vi "test.vi"() -> ()   [LabVIEW 2013]
uses:
  InfoTable.lvclass
panel:
  out "数组":cluster{"ID":dbl, "食品名称":string, "价格":dbl}[](array[cluster])
  out "Exist?":bool
  out "食品信息 2":cluster{"ID":dbl, "食品名称":string, "价格":dbl}
  in  "食品信息":cluster{"ID":dbl, "食品名称":string, "价格":dbl}
  in  "枚举":enum16{"获取", "清空", "插入", "删除", "查询"}(ring)
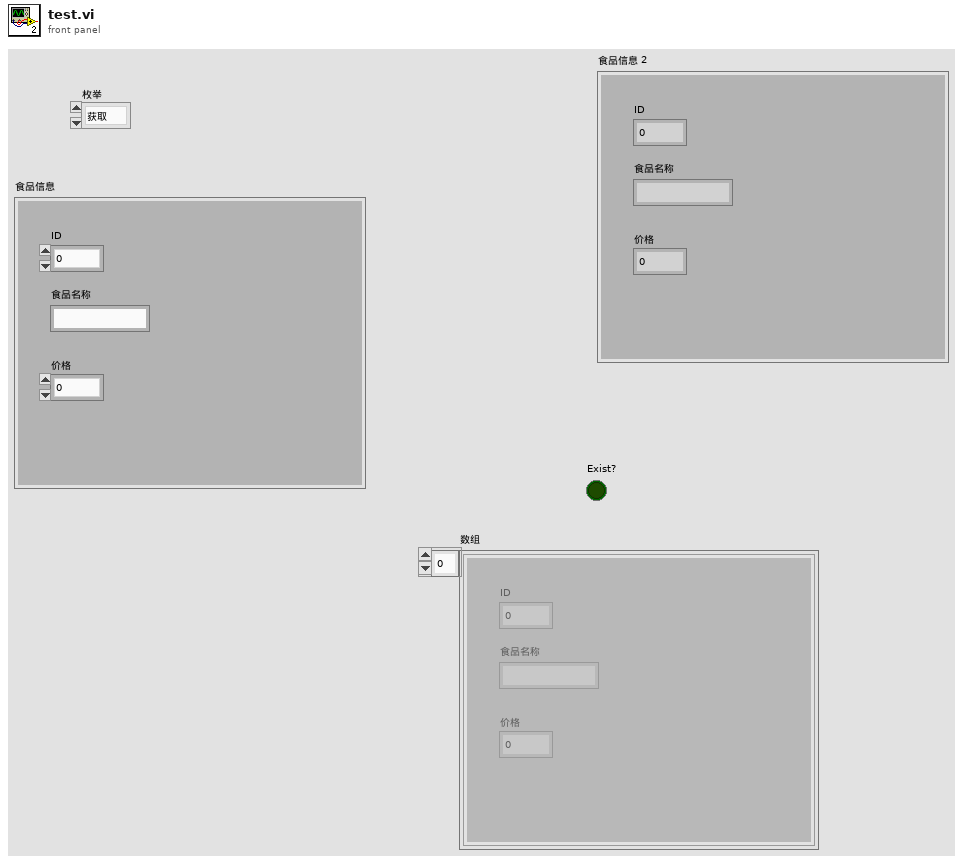
[diagram p1: front panel]
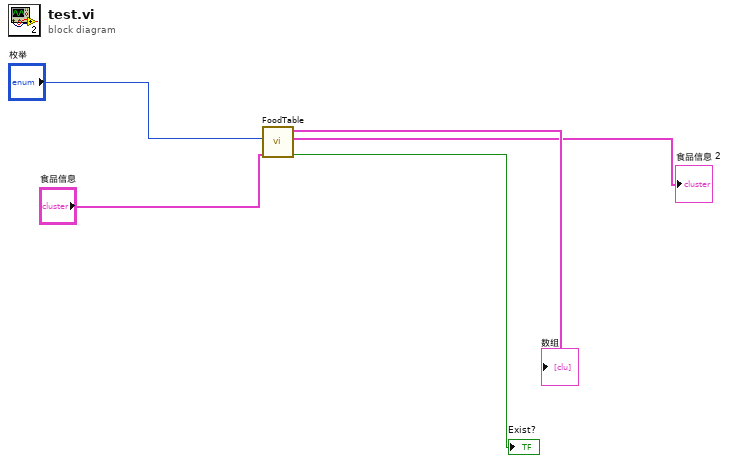
[diagram p0: block diagram]
diagram:
  n1 = call "FoodTable.vi"("食品信息"="食品信息", "枚举"="枚举") -> ("Exist?"=→"Exist?":bool, "食品信息 2"=→"食品信息 2":cluster{"ID":dbl, "食品名称":string, "价格":dbl}, "数组"=→"数组":cluster{"ID":dbl, "食品名称":string, "价格":dbl}[])  [unwired: 3 in]
